vi "saveStatetoMemento.vi"(8 "error in (no error)":errorcluster, 10 "Memento In":refnum<class "Memento.lvclass">, 11 "Originator in":refnum<class "Originator.lvclass">) -> (0 "error out":errorcluster, 2 "Memento On":refnum<class "Memento.lvclass">, 3 "Originator out":refnum<class "Originator.lvclass">)   [LabVIEW 2017, in "Originator.lvclass"]
uses:
  Originator.lvclass
  Memento Class/Memento.lvclass
  Originator.lvclass/Originator.ctl
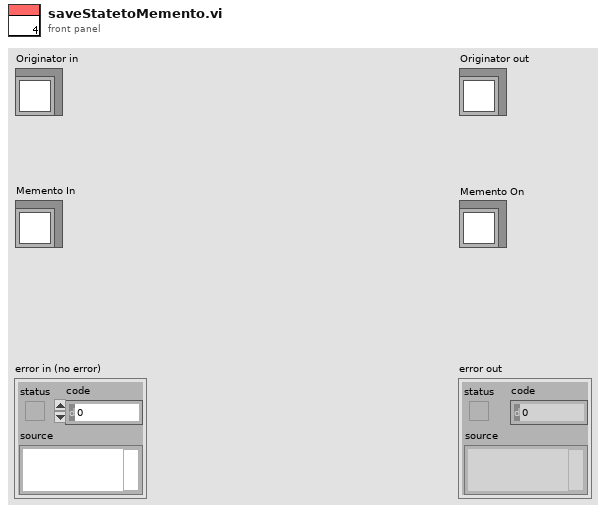
[diagram p1: front panel]
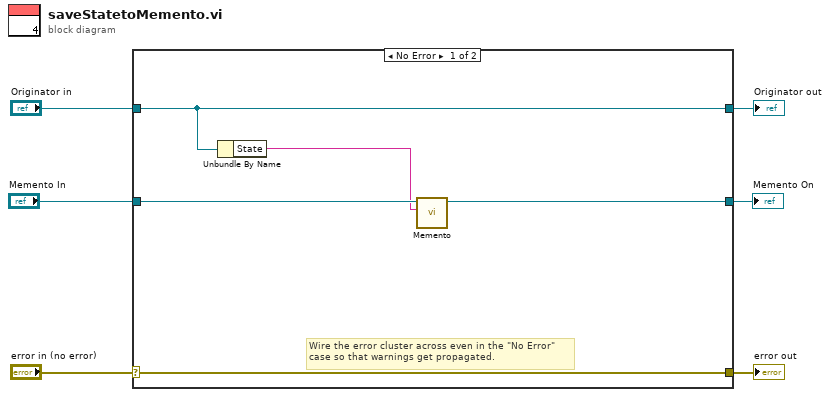
[diagram p0: block diagram]
diagram:
  n1 = case shown="No Error" "error in (no error)" {
    selector: "error in (no error)" -> [w11 w14]
    tunnel: [w11 w14] -> w5
    tunnel: [w9 w13] -> w3
    tunnel: "Originator in" -> [w9 w13]
    tunnel: "Memento In" -> [w10 w12]
    tunnel: [w8 w12] -> w1
    frame No Error {
      # "Wire the error cluster across even in the \"No Error\"\ncase so that warnings get propagated."
      n2 = Unbundle By Name(w9) -> ("State"=w7:string)
      n3 = call "Memento.vi"("State"=w7, "Memento in"=w10) -> ("Memento out"=w8:refnum<class "Memento.lvclass">)  [unwired: 8 in, 1 out]
    }
    frame Error {
    }
  }
  "error out" <- w5
  "Originator out" <- w3
  "Memento On" <- w1
